vi "read station dio map config.vi"(8 "error in":errorcluster, 10 "station idx":i32, 11 "configuration file path in":path) -> (0 "error out":errorcluster, 1 "D in map":T3, 2 "D out map":T1={"Comm Power"=enum."Sunshade Motor Relay 2", "Switch 1"=enum."Sunshade Motor Relay 2", "Switch 2"=enum."Sunshade Motor Relay 2", "Switch 3"=enum."Sunshade Motor Relay 2", "Switch 4"=enum."Sunshade Motor Relay 2", "Switch 5"=enum."Sunshade Motor Relay 2", "Switch 6"=enum."Sunshade Motor Relay 2", "Glass Analog Switch 1"=enum."Sunshade Motor Relay 2", "Glass Analog Switch 2"=enum."Sunshade Motor Relay 2", "Glass Analog Switch 3"=enum."Sunshade Motor Relay 2", "Glass Analog Switch 4"=enum."Sunshade Motor Relay 2", "Glass Motor Relay 1"=enum."Sunshade Motor Relay 2", "Glass Motor Relay 2"=enum."Sunshade Motor Relay 2", "Sunshade Motor Relay 1"=enum."Sunshade Motor Relay 2", "Sunshade Motor Relay 2"=enum."Sunshade Motor Relay 2", "Ignition High"=enum."Sunshade Motor Relay 2", "Ignition Low"=enum."Sunshade Motor Relay 2", "Battery"=enum."Sunshade Motor Relay 2", "Sunshade Analog Switch 1"=enum."Sunshade Motor Relay 2", "Sunshade Analog Switch 2"=enum."Sunshade Motor Relay 2", "Sunshade Analog Switch 3"=enum."Sunshade Motor Relay 2", "Sunshade Analog Switch 4"=enum."Sunshade Motor Relay 2", "NI LIN"=enum."Sunshade Motor Relay 2", "RS232 LIN"=enum."Sunshade Motor Relay 2", "RS232"=enum."Sunshade Motor Relay 2", "CAN"=enum."Sunshade Motor Relay 2", "Park/Enable"=enum."Sunshade Motor Relay 2", "Battery Sense"=enum."Sunshade Motor Relay 2"}, 3 "configuration file path out":path)   [LabVIEW 2018]
uses:
  02.Type Def's/station DI map.ctl
  05.UserVI's/type defs/EOL Global Digital Input Control.ctl
  02.Type Def's/station DO map.ctl
  05.UserVI's/type defs/EOL Global Digital Output Control.ctl
  05.UserVI's/file io/ini/type defs/ini file actions.ctl
  05.UserVI's/file io/ini/type defs/ini entry.ctl
  05.UserVI's/file io/ini/type defs/ini entry types.ctl
  05.UserVI's/file io/ini/type defs/ini entry value.ctl
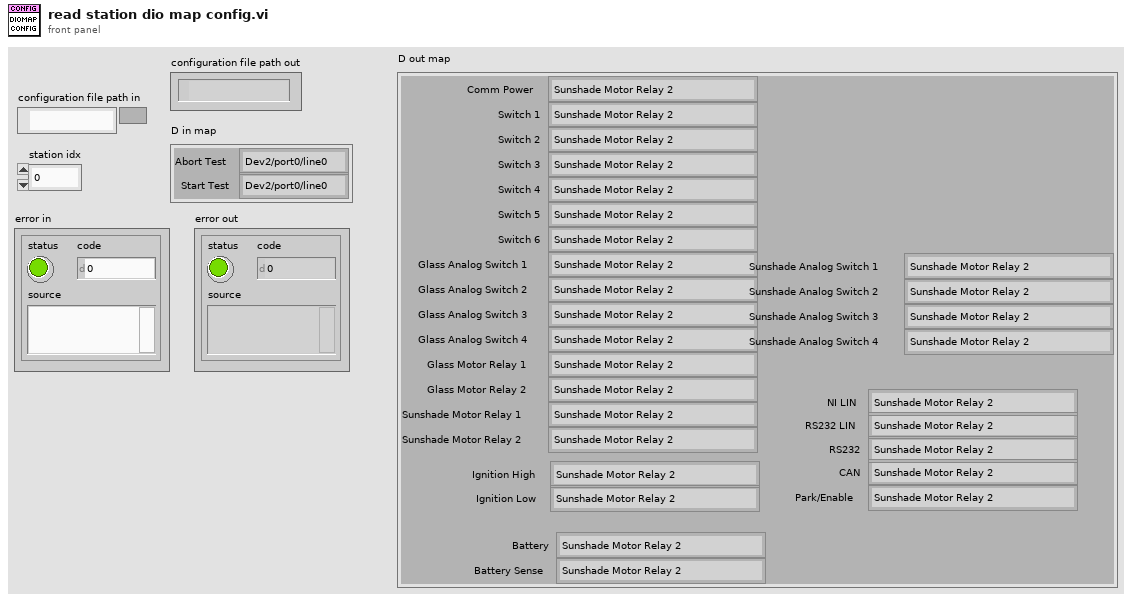
[diagram p1: front panel]
types:
  T1 = typedef "station DO map.ctl" = cluster{"Comm Power":T2, "Switch 1":T2, "Switch 2":T2, "Switch 3":T2, "Switch 4":T2, "Switch 5":T2, "Switch 6":T2, "Glass Analog Switch 1":T2, "Glass Analog Switch 2":T2, "Glass Analog Switch 3":T2, "Glass Analog Switch 4":T2, "Glass Motor Relay 1":T2, "Glass Motor Relay 2":T2, "Sunshade Motor Relay 1":T2, "Sunshade Motor Relay 2":T2, "Ignition High":T2, "Ignition Low":T2, "Battery":T2, "Sunshade Analog Switch 1":T2, "Sunshade Analog Switch 2":T2, "Sunshade Analog Switch 3":T2, "Sunshade Analog Switch 4":T2, "NI LIN":T2, "RS232 LIN":T2, "RS232":T2, "CAN":T2, "Park/Enable":T2, "Battery Sense":T2}
  T2 = typedef "EOL Global Digital Output Control.ctl" = enum16{"Battery", "IGN High", "IGN Low", "LIN", "CAN", "Switch 1", "Switch 2", "Switch 3", "Switch 4", "Switch 5", "Switch 6", "Glass Analog Switch 1", "Glass Analog Switch 2", "Glass Analog Switch 3", "Glass Analog Switch 4", "Sunshade Analog Switch 1", "Sunshade Analog Switch 2", "Sunshade Analog Switch 3", "Sunshade Analog Switch 4", "Glass Motor Relay 1", "Glass Motor Relay 2", "Sunshade Motor Relay 1", "Sunshade Motor Relay 2"}
  T3 = typedef "station DI map.ctl" = cluster{"Abort Test":T4, "Start Test":T4}
  T4 = typedef "EOL Global Digital Input Control.ctl" = enum16{"Dev2/port0/line0", "Dev2/port0/line1", "Dev2/port0/line2", "Dev2/port0/line3", "Dev2/port0/line4", "Dev2/port0/line5", "Dev2/port0/line6", "Dev2/port0/line7", "Dev2/port1/line0", "Dev2/port1/line1", "Dev2/port1/line2", "Dev2/port1/line3", "Dev2/port1/line4", "Dev2/port1/line5", "Dev2/port1/line6", "Dev2/port1/line7", "Dev2/port2/line0", "Dev2/port2/line1", "Dev2/port2/line2", "Dev2/port2/line3", "Dev2/port2/line4", "Dev2/port2/line5", "Dev2/port2/line6", "Dev2/port2/line7", "Prerun Start Test", "Prerun Abort Test", "Audit Start Test", "Audit Abort Test", "Dev2/port3/line4", "Dev2/port3/line5", "Breakin Start Test", "Breakin Abort Test", "Not Implemented"}
  T5 = typedef "ini entry.ctl" = cluster{"section":string, "key":string, "type":T6, "default value":T7}
  T6 = typedef "ini entry types.ctl" = enum16{"Boolean", "Double", "I32", "Path", "String", "U32"}
  T7 = typedef "ini entry value.ctl" = cluster{"Boolean":bool, "Dbl":dbl, "I32":i32, "Path":path, "String":string, "U32":u32}
  T8 = typedef "ini file actions.ctl" = enum16{"read ini", "write ini"}
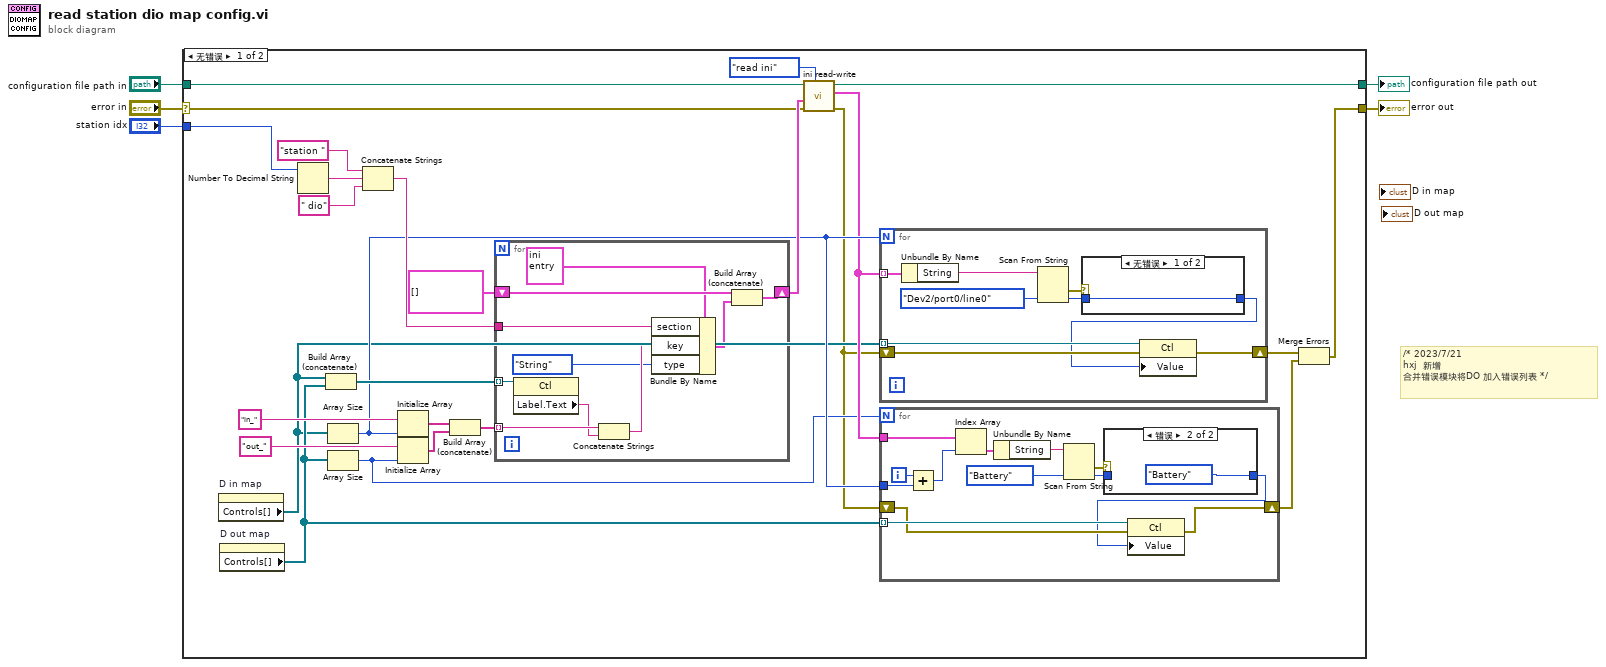
[diagram p0: block diagram]
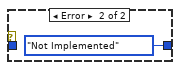
[diagram p3: hidden frame]
diagram:
  # "/* 2023/7/21\nhxj  新增\n合并错误模块将DO 加入错误列表 */"
  n1 = case shown="无错误" "error in" {
    selector: "error in" -> [w23 w69]
    tunnel: "configuration file path in" -> [w31 w68]
    tunnel: [w29 w68] -> w4
    tunnel: [w6 w69] -> w3
    tunnel: "station idx" -> [w27 _]
    frame No Error {
      n2 = property on="D in map" class="Clust (严格)"() -> ("Controls[]"=w12:refnum<vi>[])  [unwired: 2 in, 2 out]
      n3 = property on="D out map" class="Clust (严格)"() -> ("Controls[]"=w13:refnum<vi>[])  [unwired: 2 in, 2 out]
      n4 = Number To Decimal String(number=w27) -> (decimal integer string=w26:string)  [unwired: 1 in]
      n5 = Build Array (concatenate)(w12, w13) -> (w16:refnum<vi>[])
      n6 = Array Size(array=w12) -> (size(s)=w15:i32)
      n7 = Array Size(array=w13) -> (size(s)=w10:i32)
      n8 = Concatenate Strings("station ", w26, " dio") -> (w25:string)
      n9 = Initialize Array("in_", w15) -> (w19:string[])
      n10 = Initialize Array("out_", w10) -> (w18:string[])
      n11 = Build Array (concatenate)(w19, w18) -> (w17:string[])
      n12 = for {
        tunnel: w25 -> [w59]
        shift-right: [w66] -> w24
        shift-left: T5[] [] -> [w65]
        tunnel: w16 -> [w63] mode=indexing
        tunnel: w17 -> [w62] mode=indexing
        n13 = property class="Ctl"(reference=w63) -> ("Label.Text"=w61:string)  [unwired: 1 in, 2 out]
        n14 = Concatenate Strings(w62, w61) -> (w60:string)
        n15 = Bundle By Name(cluster=T5 {"section"="", "key"="", "type"=enum."Boolean", "default value"={"Boolean"=FALSE, "Dbl"=0.0, "I32"=0, "Path"=path "", "String"="", "U32"=0}}, "section"=w59, "key"=w60, "type"=ini_entry_types."String") -> (w67:T5)
        n16 = Build Array (concatenate)(w65, w67) -> (w66:T5[])
      }
      n17 = call "ini read-write.vi"("action"=ini_file_actions."read ini", "error in (no error)"=w23, "ini entry descriptors"=w24, "configuration file path"=w31) -> ("error out"=w9:errorcluster, "values out"=w14:T7[], "configuration file path out"=w29:path)  [unwired: 5 in]
      n18 = for {
        N: w15 -> [_]
        tunnel: w14 -> [w50] mode=indexing
        tunnel: w12 -> [w55] mode=indexing
        shift-right: [w54] -> w8
        shift-left: w9 -> [w53]
        n19 = Unbundle By Name(w50) -> ("String"=w52:string)
        n20 = Scan From String(input string=w52, default 1=EOL_Global_Digital_Input_Control."Dev2/port0/line0" ("Abort Test")) -> (error out=w49:errorcluster, output 1=w47:T4)  [unwired: 3 in, 2 out]
        n21 = case shown="无错误" w49 {
          tunnel: [w56 EOL_Global_Digital_Input_Control."Not Implemented" ("Abort Test")] -> w48
          tunnel: w47 -> [w56 _]
          frame No Error {
          }
          frame Error {
          }
        }
        n22 = property class="Ctl"(reference=w55, error in=w53, "Value"=w48) -> (error out=w54:errorcluster)  [unwired: 1 out]
      }
      n23 = for {
        N: w10 -> [_]
        tunnel: w14 -> [w44]
        tunnel: w13 -> [w42] mode=indexing
        shift-right: [w41] -> w7
        shift-left: w9 -> [w40]
        tunnel: w15 -> [w35]
        i -> [w36]
        n24 = Add(x=w36, y=w35) -> (x+y=w37:i32)
        n25 = Index Array(array=w44, index=w37) -> (element=w43:T7)
        n26 = Unbundle By Name(w43) -> ("String"=w38:string)
        n27 = Scan From String(input string=w38, default 1=EOL_Global_Digital_Output_Control."Battery" ("Glass Analog Switch 4")) -> (error out=w34:errorcluster, output 1=w32:T2)  [unwired: 3 in, 2 out]
        n28 = case shown="错误" w34 {
          tunnel: [w45 EOL_Global_Digital_Output_Control."Battery" ("Glass Analog Switch 4")] -> w33
          tunnel: w32 -> [w45 _]
          frame No Error {
          }
          frame Error {
          }
        }
        n29 = property class="Ctl"(reference=w42, error in=w40, "Value"=w33) -> (error out=w41:errorcluster)  [unwired: 1 out]
      }
      n30 = Merge Errors(w8, w7) -> (w6:errorcluster)
    }
    frame Error {
    }
  }
  "configuration file path out" <- w4
  "error out" <- w3
